vi "Autocomplete Options.vi"(11 "ElementEditorPanel in":refnum<class "ElementEditorPanel.lvclass">) -> (2 "Autocomplete Options":refnum<class "Shared Options.lvclass">)   [LabVIEW 2020, in "VolatusGUIControls.lvlib" / "ElementEditorPanel.lvclass"]
uses:
  ElementEditorPanel.lvclass
  ElementEditorPanel.lvclass/ElementEditorPanel.ctl
  lv-autocomplete/AutoComplete/Shared Options/Shared Options.lvclass
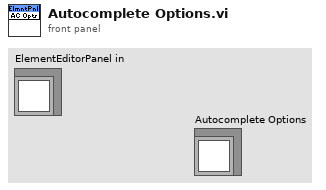
[diagram p1: front panel]
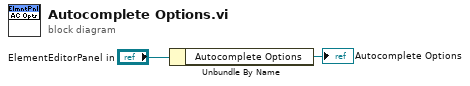
[diagram p0: block diagram]
diagram:
  n1 = Unbundle By Name("ElementEditorPanel in") -> ("Autocomplete Options"=→"Autocomplete Options":refnum<class "Shared Options.lvclass">)
